vi "JLINKARM Is Connected.vi"(8 "error in (no error)":errorcluster caption="错误输入（无错误）") -> (0 "error out":errorcluster caption="错误输出", 3 "function return":i32)   [LabVIEW 2016, in "JLinkARM.lvlib"]
doc: "int JLINKARM_IsConnected(void)"
uses:
  <userlib>/LV-JLinkARM/JLinkARM.lvlib
  <userlib>/LV-JLinkARM/JLinkARM.dll
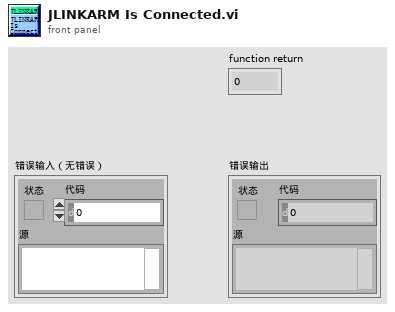
[diagram p1: front panel]
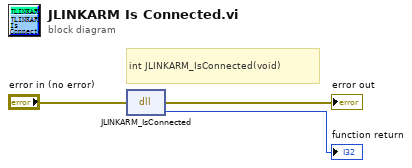
[diagram p0: block diagram]
diagram:
  # "int JLINKARM_IsConnected(void)"
  n1 = dll-call lib="C:/Program Files (x86)/National Instruments/LabVIEW 2016/user.lib/LV-JLinkARM/JLinkARM.*" fn="JLINKARM_IsConnected"(error in="error in (no error)") -> (error out=→"error out":errorcluster, →"function return":i32)  [unwired: 2 in, 1 out]
